vi "ReadStringRegister.vi"(8 "index":i32, 10 "Snpx":refnum<k24>, 11 "error in":errorcluster) -> (0 "Value":string, 3 "error out":errorcluster)   [LabVIEW 2016, in "UnderAutomation.Fanuc.lvlib"]
uses:
  UnderAutomation.Fanuc.lvlib
  C:/Users/fg/Documents/Fanuc.vi/LabVIEW_2024/UnderAutomation.Fanuc/lib/UnderAutomation.Fanuc.dll
  LabVIEW_2024/UnderAutomation.Fanuc/lib/UnderAutomation.Fanuc.dll
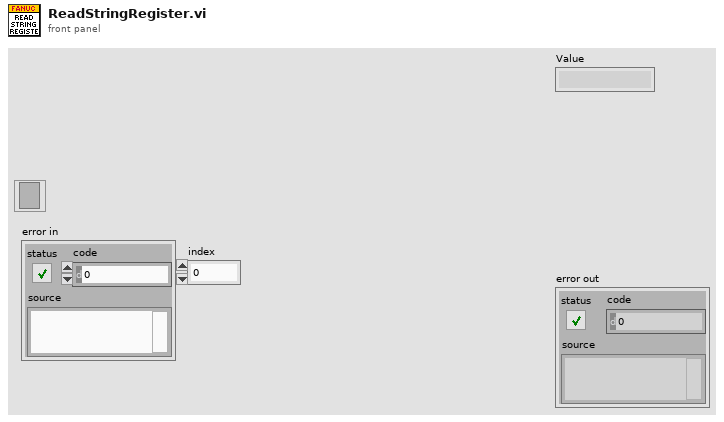
[diagram p1: front panel]
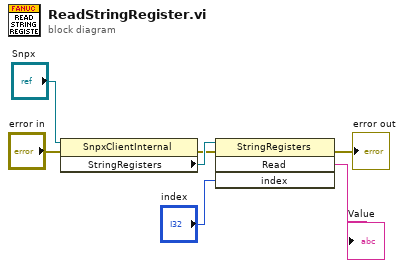
[diagram p0: block diagram]
diagram:
  n1 = property class="SnpxClientInternal"(reference="Snpx", error in="error in") -> (error out=w4:errorcluster, "StringRegisters"=w5:refnum<k24>)  [unwired: 1 out]
  n2 = invoke class="StringRegisters" method="Read"(reference=w5, error in=w4, "index"="index") -> (error out=→"error out":errorcluster, "Read"=→"Value":string)  [unwired: 1 in, 2 out]
